vi "Match Info With Write.vi"(0 "Game Data":string, 1 "Colour":enum16{"Blue", "Red"}(ring)) -> (2 "Our Switch (R)":u32(colorbox), 3 "Our Switch (L)":u32(colorbox), 4 "Other Switch (R)":u32(colorbox), 5 "Other Switch (L)":u32(colorbox), 6 "Scale (L)":u32(colorbox), 7 "Scale (R)":u32(colorbox))   [LabVIEW 2017]
uses:
  <vilib>/Rock Robotics/Network Tables/NT Write Number.vi
panel:
  # "FAR SWITCH"
  # "SCALE"
  # "OUR SWITCH"
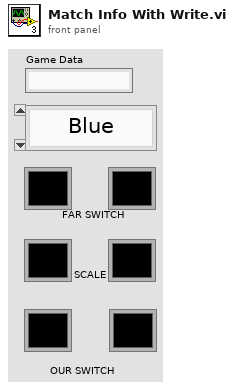
[diagram p1: front panel]
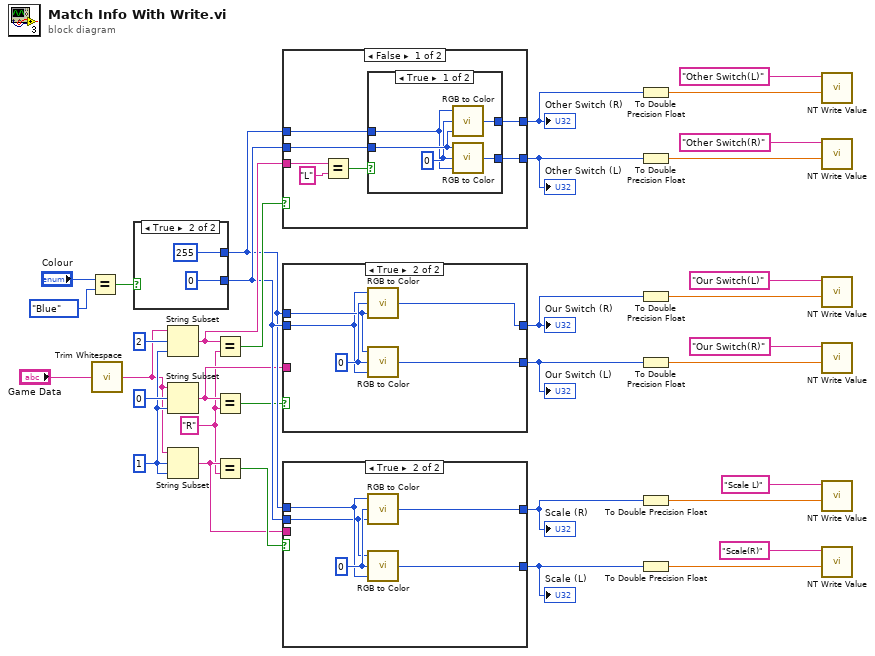
[diagram p0: block diagram]
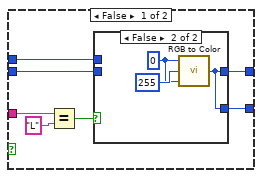
[diagram p2: hidden frame]
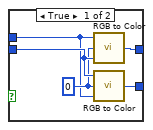
[diagram p3: hidden frame]
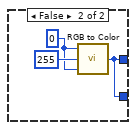
[diagram p4: hidden frame]
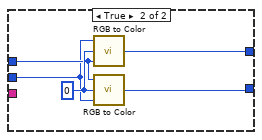
[diagram p5: hidden frame]
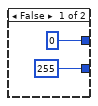
[diagram p6: hidden frame]
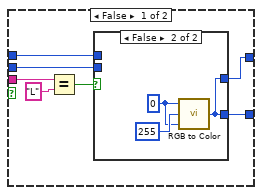
[diagram p7: hidden frame]
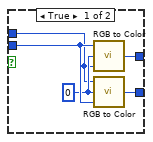
[diagram p8: hidden frame]
diagram:
  w1 = "R" ("y")
  w32 = 1 ("length (rest)")
  n1 = Equal?(x="Colour", y=enum16{"Blue", "Red"}."Blue") -> (x = y?=w27:bool)
  n2 = call <vilib>:"Trim Whitespace.vi"("string"="Game Data") -> ("trimmed string"=w30:string)  [unwired: 1 in]
  n3 = case shown="True" w27 {
    tunnel: [u8 0 ("R") u8 255 ("R")] -> w23
    tunnel: [u8 255 ("R") u8 0 ("R")] -> w24
    frame False {
    }
    frame True {
    }
  }
  n4 = String Subset(string=w30, offset (0)=2, length (rest)=w32) -> (substring=w26:string)
  n5 = String Subset(string=w30, offset (0)=0, length (rest)=w32) -> (substring=w22:string)
  n6 = String Subset(string=w30, offset (0)=w32, length (rest)=w32) -> (substring=w33:string)
  n7 = Equal?(x=w26, y=w1) -> (x = y?=w25:bool)
  n8 = Equal?(x=w22, y=w1) -> (x = y?=w21:bool)
  n9 = Equal?(x=w33, y=w1) -> (x = y?=w34:bool)
  n10 = case shown="False" w25 {
    tunnel: [w43 w59] -> w17
    tunnel: w26 -> [w45 _]
    tunnel: w24 -> [w42 w55]
    tunnel: w23 -> [w41 w56]
    tunnel: [w40 w57] -> w19
    frame False {
      n11 = Equal?(x=w45, y="L") -> (x = y?=w46:bool)
      n12 = case shown="True" w46 {
        tunnel: [w48 w52] -> w43
        tunnel: w42 -> [w51 _]
        tunnel: w41 -> [w49 _]
        tunnel: [w47 w52] -> w40
        frame True {
          w50 = u8 0 ("B")
          n13 = call <vilib>:"RGB to Color.vi"("B"=w51, "G"=w50, "R"=w49) -> ("Color"=w48:u32)
          n14 = call <vilib>:"RGB to Color.vi"("B"=w49, "G"=w50, "R"=w51) -> ("Color"=w47:u32)
        }
        frame False {
          w53 = u8 0 ("B")
          n15 = call <vilib>:"RGB to Color.vi"("B"=w53, "G"=u8 255 ("R"), "R"=w53) -> ("Color"=w52:u32)
        }
      }
    }
    frame True {
      w58 = u8 0 ("B")
      n16 = call <vilib>:"RGB to Color.vi"("B"=w56, "G"=w58, "R"=w55) -> ("Color"=w59:u32)
      n17 = call <vilib>:"RGB to Color.vi"("B"=w55, "G"=w58, "R"=w56) -> ("Color"=w57:u32)
    }
  }
  "Other Switch (R)" <- w17
  "Other Switch (L)" <- w19
  n18 = case shown="True" w21 {
    tunnel: [w63 w79] -> w5
    tunnel: w22 -> [w65 _]
    tunnel: w24 -> [w62 w75]
    tunnel: w23 -> [w61 w76]
    tunnel: [w60 w77] -> w4
    frame False {
      n19 = Equal?(x=w65, y="L") -> (x = y?=w66:bool)
      n20 = case shown="False" w66 {
        tunnel: [w68 w72] -> w63
        tunnel: w62 -> [w71 _]
        tunnel: w61 -> [w69 _]
        tunnel: [w67 w72] -> w60
        frame True {
          w70 = u8 0 ("B")
          n21 = call <vilib>:"RGB to Color.vi"("B"=w71, "G"=w70, "R"=w69) -> ("Color"=w68:u32)
          n22 = call <vilib>:"RGB to Color.vi"("B"=w69, "G"=w70, "R"=w71) -> ("Color"=w67:u32)
        }
        frame False {
          w73 = u8 0 ("B")
          n23 = call <vilib>:"RGB to Color.vi"("B"=w73, "G"=u8 255 ("R"), "R"=w73) -> ("Color"=w72:u32)
        }
      }
    }
    frame True {
      w78 = u8 0 ("B")
      n24 = call <vilib>:"RGB to Color.vi"("B"=w76, "G"=w78, "R"=w75) -> ("Color"=w79:u32)
      n25 = call <vilib>:"RGB to Color.vi"("B"=w75, "G"=w78, "R"=w76) -> ("Color"=w77:u32)
    }
  }
  "Our Switch (R)" <- w5
  "Our Switch (L)" <- w4
  n26 = case shown="True" w34 {
    tunnel: [w83 w99] -> w2
    tunnel: w33 -> [w85 _]
    tunnel: w24 -> [w82 w95]
    tunnel: w23 -> [w81 w96]
    tunnel: [w80 w97] -> w3
    frame False {
      n27 = Equal?(x=w85, y="L") -> (x = y?=w86:bool)
      n28 = case shown="False" w86 {
        tunnel: [w88 w92] -> w83
        tunnel: w82 -> [w91 _]
        tunnel: w81 -> [w89 _]
        tunnel: [w87 w92] -> w80
        frame True {
          w90 = u8 0 ("B")
          n29 = call <vilib>:"RGB to Color.vi"("B"=w89, "G"=w90, "R"=w91) -> ("Color"=w87:u32)
          n30 = call <vilib>:"RGB to Color.vi"("B"=w91, "G"=w90, "R"=w89) -> ("Color"=w88:u32)
        }
        frame False {
          w93 = u8 0 ("B")
          n31 = call <vilib>:"RGB to Color.vi"("B"=w93, "G"=u8 255 ("R"), "R"=w93) -> ("Color"=w92:u32)
        }
      }
    }
    frame True {
      w98 = u8 0 ("B")
      n32 = call <vilib>:"RGB to Color.vi"("B"=w95, "G"=w98, "R"=w96) -> ("Color"=w97:u32)
      n33 = call <vilib>:"RGB to Color.vi"("B"=w96, "G"=w98, "R"=w95) -> ("Color"=w99:u32)
    }
  }
  "Scale (L)" <- w2
  "Scale (R)" <- w3
  n34 = To Double Precision Float(number=w17) -> (double precision float=w16:dbl)
  n35 = To Double Precision Float(number=w19) -> (double precision float=w18:dbl)
  n36 = To Double Precision Float(number=w5) -> (double precision float=w11:dbl)
  n37 = To Double Precision Float(number=w4) -> (double precision float=w10:dbl)
  n38 = To Double Precision Float(number=w3) -> (double precision float=w8:dbl)
  n39 = To Double Precision Float(number=w2) -> (double precision float=w9:dbl)
  n40 = call-poly <vilib>:"NT Write Value.vi"("Numeric"=w16, "Name"="Other Switch(L)") -> ()  [unwired: 9 in, 1 out]
  n41 = call-poly <vilib>:"NT Write Value.vi"("Numeric"=w18, "Name"="Other Switch(R)") -> ()  [unwired: 9 in, 1 out]
  n42 = call-poly <vilib>:"NT Write Value.vi"("Numeric"=w11, "Name"="Our Switch(L)") -> ()  [unwired: 9 in, 1 out]
  n43 = call-poly <vilib>:"NT Write Value.vi"("Numeric"=w10, "Name"="Our Switch(R)") -> ()  [unwired: 9 in, 1 out]
  n44 = call-poly <vilib>:"NT Write Value.vi"("Numeric"=w8, "Name"="Scale L)") -> ()  [unwired: 9 in, 1 out]
  n45 = call-poly <vilib>:"NT Write Value.vi"("Numeric"=w9, "Name"="Scale(R)") -> ()  [unwired: 9 in, 1 out]
